vi "Read JSONPayload.vi"(8 "error in (no error)":errorcluster, 11 "JSONPacket in":refnum<class "JSONPacket.lvclass">) -> (0 "error out":errorcluster, 2 "JSONPayload.lvclass":refnum<class "JSONPayload.lvclass">, 3 "JSONPacket out":refnum<class "JSONPacket.lvclass">)   [LabVIEW 2019, in "JSONPacket.lvclass"]
uses:
  JSONPacket.lvclass
  JSONPayload/JSONPayload.lvclass
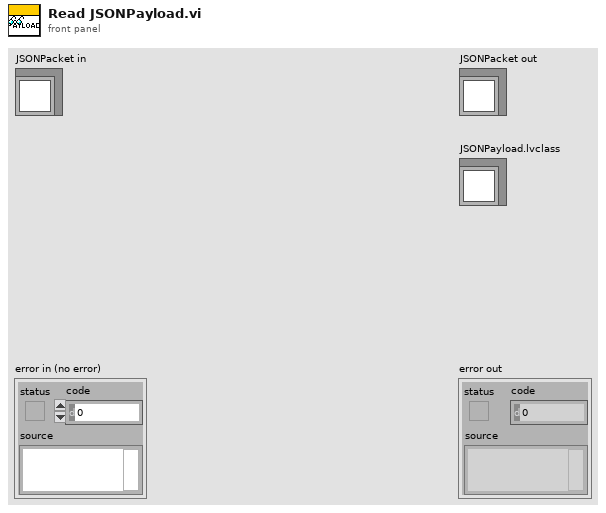
[diagram p1: front panel]
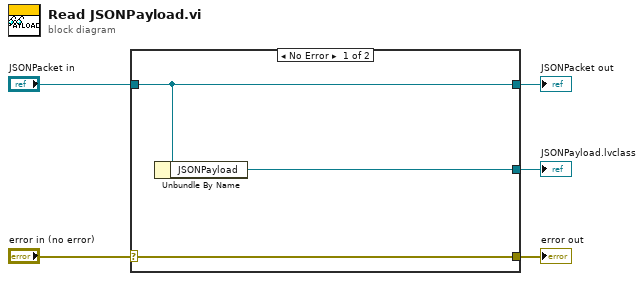
[diagram p0: block diagram]
diagram:
  n1 = case shown="No Error" "error in (no error)" {
    selector: "error in (no error)" -> [w8 w9]
    tunnel: [w8 w9] -> w4
    tunnel: [w7 w10] -> w2
    tunnel: "JSONPacket in" -> [w7 w10]
    tunnel: [w6 _] -> w1
    frame No Error {
      n2 = Unbundle By Name(w7) -> ("JSONPayload"=w6:refnum<class "JSONPayload.lvclass">)
    }
    frame Error {
    }
  }
  "error out" <- w4
  "JSONPacket out" <- w2
  "JSONPayload.lvclass" <- w1
